vi "Read Time.vi"(8 "error in (no error)":errorcluster, 11 "ControlMouseLeaveMsg in":refnum<class "ControlMouseLeaveMsg.lvclass">) -> (0 "error out":errorcluster, 2 "Time":u32, 3 "ControlMouseLeaveMsg out":refnum<class "ControlMouseLeaveMsg.lvclass">)   [LabVIEW 2020, in "MVA Framework.lvlib" / "ActorEvents.lvlib" / "ControlMouseLeaveMsg.lvclass"]
uses:
  ControlMouseLeaveMsg.lvclass
  ControlMouseLeaveMsg.lvclass/ControlMouseLeaveMsg.ctl
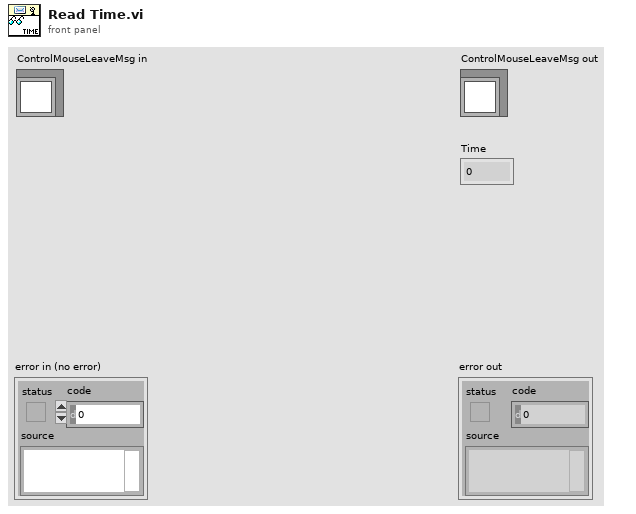
[diagram p1: front panel]
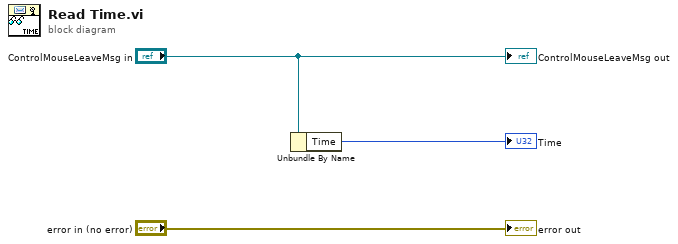
[diagram p0: block diagram]
diagram:
  n1 = Unbundle By Name("ControlMouseLeaveMsg in") -> ("Time"=→"Time":u32)
  "error out" <- "error in (no error)"
  "ControlMouseLeaveMsg out" <- "ControlMouseLeaveMsg in"
